vi "MotionProfiles_UpdateTalonMode.vi"(8 "error in (no error)":errorcluster, 10 "Talon Control Mode":T1, 11 "MotionProfiles in":refnum<class "MotionProfiles.lvclass">) -> (0 "error out":errorcluster, 3 "MotionProfiles out":refnum<class "MotionProfiles.lvclass">)   [LabVIEW 2016]
uses:
  MotionProfiles.lvclass
  <vilib>/Rock Robotics/WPI/ThirdParty/CanMotor/TalonSRX/WPI_CANTalonSRX_APIControlMode.ctl
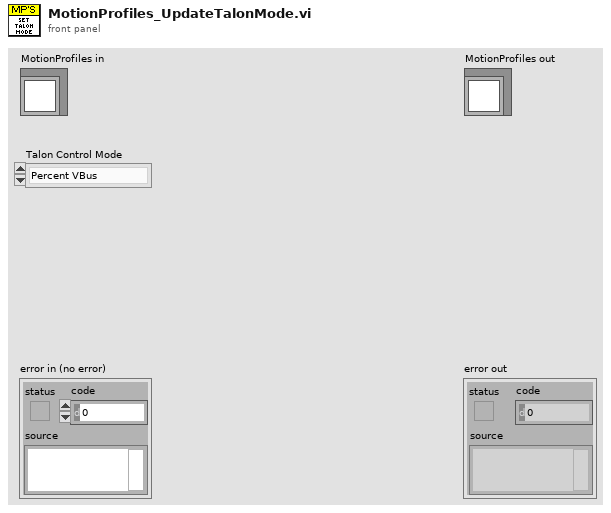
[diagram p1: front panel]
types:
  T1 = typedef "WPI_CANTalonSRX_APIControlMode.ctl" = enum8{"Percent VBus", "Speed", "Position", "Slave", "Unchanged / Invalid", "Voltage Compensation", "Current", "Motion Profile", "Motion Magic"}
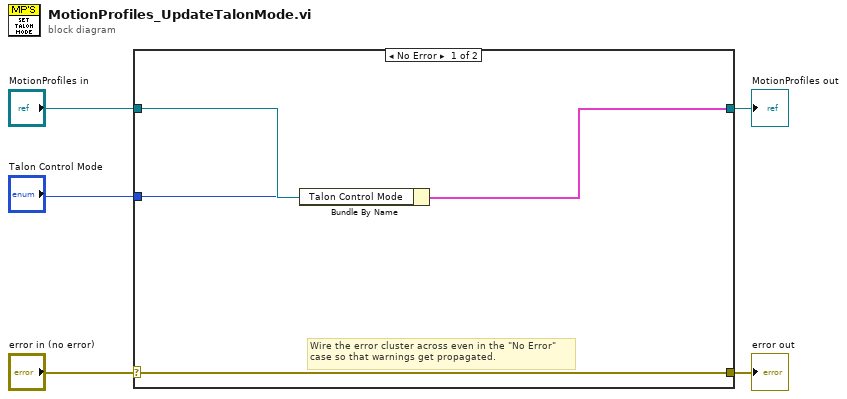
[diagram p0: block diagram]
diagram:
  n1 = case shown="No Error" "error in (no error)" {
    selector: "error in (no error)" -> [w9 w11]
    tunnel: [w9 w11] -> w4
    tunnel: [w7 w10] -> w2
    tunnel: "MotionProfiles in" -> [w8 w10]
    tunnel: "Talon Control Mode" -> [w6 _]
    frame No Error {
      # "Wire the error cluster across even in the \"No Error\"\ncase so that warnings get propagated."
      n2 = Bundle By Name(cluster=w8, "Talon Control Mode"=w6) -> (w7:cluster{})
    }
    frame Error {
    }
  }
  "error out" <- w4
  "MotionProfiles out" <- w2
